vi "2일차11vi.vi"() -> ()   [LabVIEW 2014]
panel:
  out "부분배열 2":i32[](array[numeric])
  out "부분배열":i32[](array[numeric])
  out "원소":i32
  out "배열":i32[][](array[numeric])
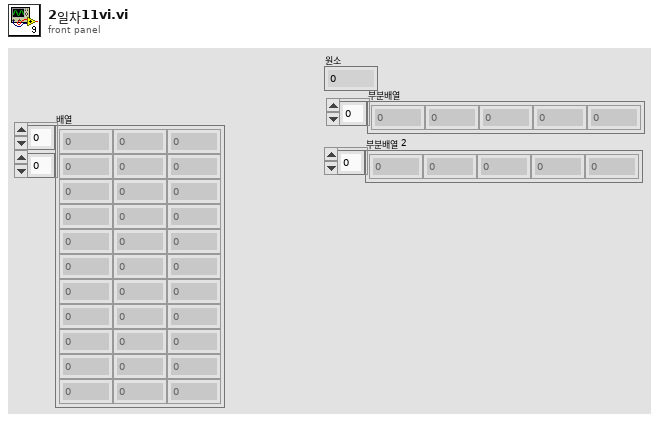
[diagram p1: front panel]
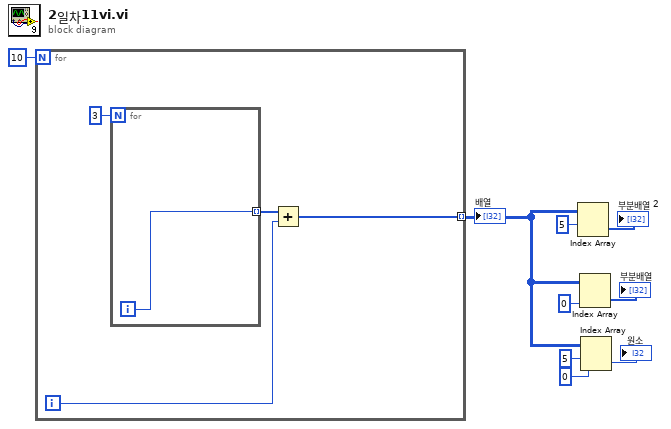
[diagram p0: block diagram]
diagram:
  n1 = for {
    N: 10 -> [_]
    tunnel: [w10] -> w1 mode=indexing
    i -> [w12]
    n2 = for {
      N: 3 -> [_]
      tunnel: [w14] -> w11 mode=indexing
      i -> [w14]
    }
    n3 = Add(x=w11, y=w12) -> (x+y=w10:i32[])
  }
  "배열" <- w1
  n4 = Index Array(array=w1, index (row)=5 ("인덱스 (행)")) -> (element=→"부분배열 2":i32[])  [unwired: 1 in]
  n5 = Index Array(array=w1, index (col)=0 ("비활성화된 인덱스 (열)")) -> (element=→"부분배열":i32[])  [unwired: 1 in]
  n6 = Index Array(array=w1, index (row)=5 ("인덱스 (행)"), index (col)=0 ("비활성화된 인덱스 (열)")) -> (element=→"원소":i32)
